vi "sem_destroy.vi"(8 "error in (no error)":errorcluster, 11 "sempahore ptr in":u64) -> (0 "error out":errorcluster, 3 "semaphore ptr out":u64)   [LabVIEW 2016, in "Linux RT IPC.POSIX Threads.lvlib" / "POSIX Thread Object.lvclass"]
uses:
  POSIX Thread Object.lvclass
  Controls/pthread functions.ctl
  <vilib>/NI/NI Linux RT Errno/Linux Errno.lvlib
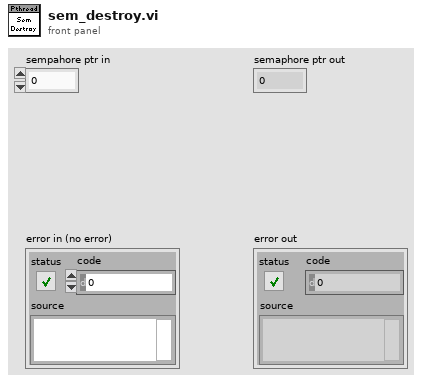
[diagram p1: front panel]
types:
  T1 = typedef "Linux RT IPC.POSIX Threads.lvlib/POSIX Thread Object.lvclass/pthread functions.ctl" = enum16{"unspecified", "pthread_condattr_init", "pthread_condattr_destroy", "pthread_condattr_getclock", "pthread_condattr_setclock", "pthread_condattr_getpshared", "pthread_condattr_setpshared", "pthread_cond_init", "pthread_cond_destroy", "pthread_cond_broadcast", "pthread_cond_signal", "pthread_cond_timedwait", "pthread_cond_wait", "pthread_mutexattr_init", "pthread_mutexattr_destroy", "pthread_mutexattr_getprioceiling", "pthread_mutexattr_setprioceiling", "pthread_mutexattr_getprotocol", "pthread_mutexattr_setprotocol", "pthread_mutexattr_getpshared", "pthread_mutexattr_setpshared", "pthread_mutexattr_gettype", "pthread_mutexattr_settype", "pthread_mutex_init", "pthread_mutex_destroy", "pthread_mutex_getprioceiling", "pthread_mutex_setprioceiling", "pthread_mutex_lock", "pthread_mutex_timedlock", "pthread_mutex_trylock", "pthread_mutex_unlock", "sem_destroy", "sem_getvalue", "sem_init", "sem_post", "sem_timedwait", "sem_trywait", "sem_wait", "barrier_init", "barrier_destroy", "barrier_wait", "barrierattr_init", "barrierattr_destroy", "barrierattr_getpshared", "barrierattr_setpshared"}
  T2 = typedef "Linux Errno.lvlib/errno.ctl" = enum16{"NO ERROR", "EPERM", "ENOENT", "ESRCH", "EINTR", "EIO", "ENXIO", "E2BIG", "ENOEXEC", "EBADF", "ECHILD", "EAGAIN", "ENOMEM", "EACCES", "EFAULT", "ENOTBLK", "EBUSY", "EEXIST", "EXDEV", "ENODEV", "ENOTDIR", "EISDIR", "EINVAL", "ENFILE", "EMFILE", "ENOTTY", "ETXTBSY", "EFBIG", "ENOSPC", "ESPIPE", "EROFS", "EMLINK", "EPIPE", "EDOM", "ERANGE", "EDADLK", "ENAMETOOLONG", "ENOLCK", "ENOSYS", "ENOTEMPTY", "ELOOP", "EWOULDBLOCK", "ENOMSG", "EIDRM", "ECHRNG", "EL2NSYNC", "EL3HLT", "EL3RST", "ELNRNG", "EUNATCH", "ENOCSI", "EL2HLT", "EBADE", "EBADR", "EXFULL", "ENOANO", "EBADRQC", "EBADSLT", "EDEADLOCK", "EBFONT", "ENOSTR", "ENODATA", "ETIME", "ENOSR", "ENONET", "ENOPKG", "EREMOTE", "ENOLINK", "EADV", "ESRMNT", "ECOMM", "EPROTO", "EMULTIHOP", "EDOTDOT", "EBADMSG", "EOVERFLOW", "ENOTUNIQ", "EBADFD", "EREMCHG", "ELIBACC", "ELIBBAD", "ELIBSCN", "ELIBMAX", "ELIBEXEC", "ELISEQ", "ERESTART", "ESTRPIPE", "EUSERS", "ENOTSOCK", "EDESTADDRREQ", "EMSGSIZE", "EPROTOTYPE", "ENOPROTOOPT", "EPROTONOSUPPORT", "ESOCKTNOSUPPORT", "EOPNOTSUPP", "EPFNOSUPPORT", "EAFNOSUPPORT", "EADDRINUSE", "EADDRNOTAVAIL", "ENETDOWN", "ENETUNREACH", "ENETRESET", "ECONNABORTED", "ECONNRESET", "ENOBUFS", "EISCONN", "ENOTCONN", "ESHUTDOWN", "ETOOMANYREFS", "ETIMEDOUT", "ECONNREFUSED", "EHOSTDOWN", "EHOSTUNREACH", "EALREADY", "EINPROGRESS", "ESTALE", "EUCLEAN", "ENOTNAM", "ENAVAIL", "EISNAM", "EREMOTEIO", "EDQUOT", "ENOMEDIUM", "EMEDIUMTYPE", "ECANCELED", "ENOKEY", "EKEYEXPIRED", "EKEYREVOKED", "EKEYREJECTED", "EOWNERDEAD", "ENOTRECOVERABLE", "ERFKILL", "EHWPOISON", "UNDEFINED"}
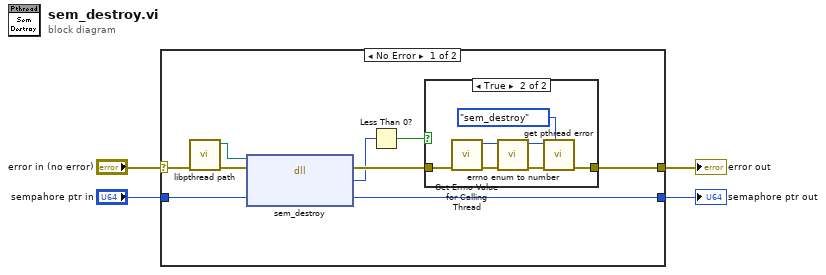
[diagram p0: block diagram]
diagram:
  n1 = case shown="No Error" "error in (no error)" {
    selector: "error in (no error)" -> [w13 w23]
    tunnel: "sempahore ptr in" -> [w12 w22]
    tunnel: [w5 w23] -> w2
    tunnel: [w11 w22] -> w1
    frame No Error {
      n2 = call "libpthread path.vi"("error in (no error)"=w13) -> ("error out"=w9:errorcluster, "path to libpthread"=w10:path)  [unwired: 9 in]
      n3 = dll-call lib="?" fn="sem_destroy"(path in=w10, error in=w9, "sem"=w12) -> (error out=w7:errorcluster, "errno"=w6:i32, "sem"=w11:u64)  [unwired: 1 in, 1 out]
      n4 = Less Than 0?(x=w6) -> (x < 0?=w8:bool)
      n5 = case shown="True" w8 {
        tunnel: w7 -> [w14 w21]
        tunnel: [w14 w19] -> w5
        frame False {
        }
        frame True {
          n6 = call <vilib>:"Get Errno Value for Calling Thread.vi"("error in (no error)"=w21) -> ("error out"=w18:errorcluster, "errno"=w17:T2)  [unwired: 9 in]
          n7 = call <vilib>:"errno enum to number.vi"("error in (no error)"=w18, "errno enum"=w17) -> ("error out"=w15:errorcluster, "errno number"=w16:i32)  [unwired: 8 in]
          n8 = call "get pthread error.vi"("function"=pthread_functions."sem_destroy", "error in (no error)"=w15, "errno"=w16) -> ("error out"=w19:errorcluster)  [unwired: 8 in]
        }
      }
    }
    frame Error {
    }
  }
  "error out" <- w2
  "semaphore ptr out" <- w1
